vi "SplitSignals.vi"(0 "VI reference":refnum<vi>, 1 "Filename":path=path "E:/LabVIEW/Data/Test Data/Subj-Austin_Trial-1_Condition-None.lvm", 11 "Error In":errorcluster) -> (2 "EGG":dynamicdata(graph), 3 "Filename Out":path=path "E:/LabVIEW/Data/Test Data/Subj-Austin_Trial-1_Condition-None.lvm" caption="Filename", 4 "Flow":dynamicdata(graph), 6 "Pressure":dynamicdata(graph), 8 "Audio":dynamicdata(graph), 10 "SPL":dynamicdata(graph), 14 "Upper SPL":dbl, 15 "Error Out":errorcluster)   [LabVIEW 2019, in "AnalysisSupport.lvlib"]
uses:
  AnalysisSupport.lvlib
panel:
  out "Signals (Array)":string[](array[string])
  out "Comment":string
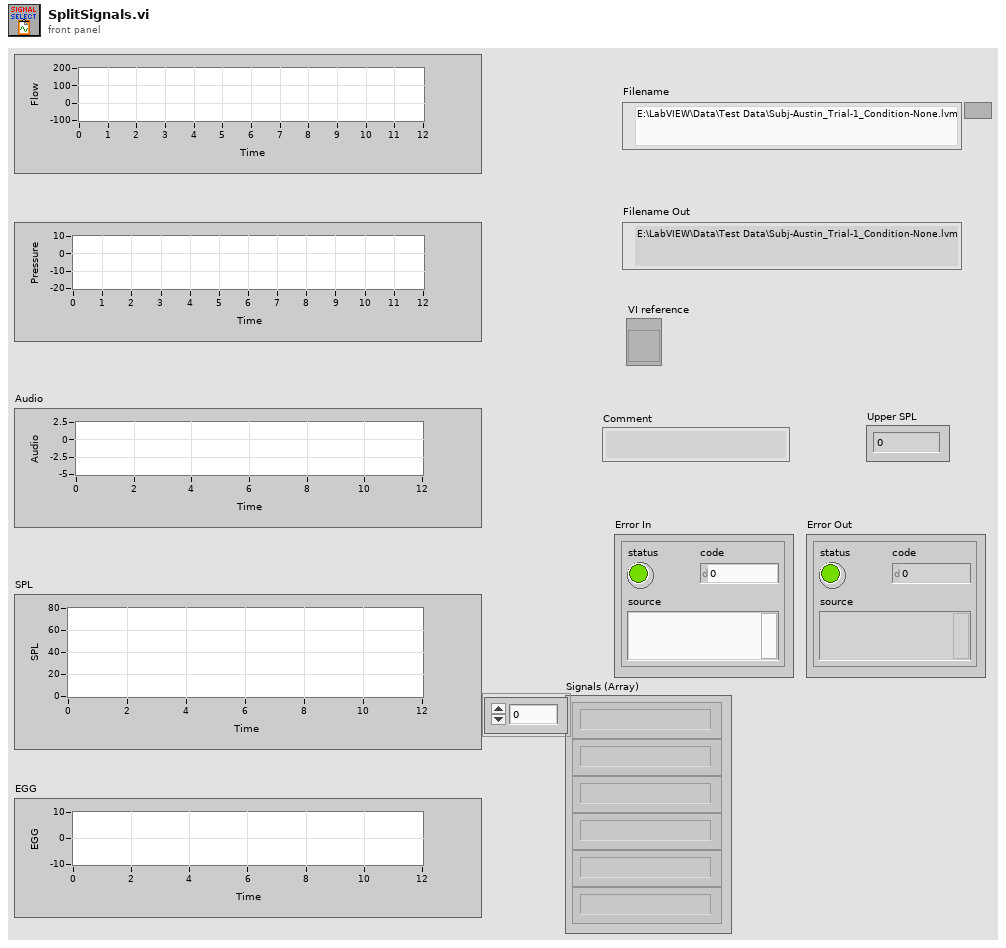
[diagram p1: front panel]
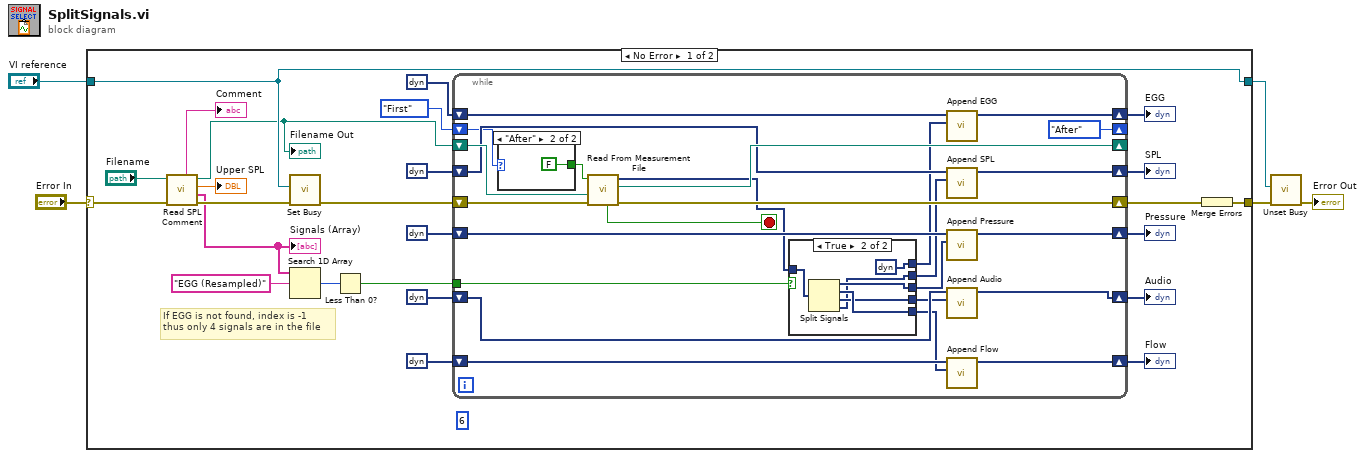
[diagram p0: block diagram]
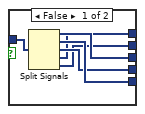
[diagram p2: hidden frame]
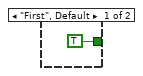
[diagram p3: hidden frame]
diagram:
  n1 = case shown="No Error" "Error In" {
    selector: "Error In" -> [w9 w71]
    tunnel: [w30 w71] -> w4
    tunnel: "VI reference" -> [w18 w70]
    tunnel: [w18 w70] -> w1
    frame No Error {
      (unwired) 6
      # "If EGG is not found, index is -1\nthus only 4 signals are in the file"
      n2 = call "Read SPL Comment.vi"("error in (no error)"=w9, "Filename"="Filename") -> ("error out"=w10:errorcluster, "Signals"=w6:string[], "Upper SPL"=→"Upper SPL":dbl, "Filename Out"=w14:path, "Comment"=→"Comment":string)  [unwired: 5 in]
      "Filename Out" <- w14
      "Signals (Array)" <- w6
      n3 = call <vilib>:"Set Busy.vi"("error in (no error)"=w10, "VI reference (current VI)"=w18) -> ("error out"=w7:errorcluster)  [unwired: 8 in, 1 out]
      n4 = Search 1D Array(1D array=w6, element="EGG (Resampled)") -> (index of element=w12:i32)  [unwired: 1 in]
      n5 = Less Than 0?(x=w12) -> (x < 0?=w11:bool)
      n6 = while {
        shift-right: [w54] -> w22
        shift-left: w7 -> [w53]
        shift-right: [w55] -> _
        shift-left: w14 -> [w52]
        shift-right: [w43] -> w25
        shift-left: dynamicdata [] ("Waveform Graph") -> [w50]
        shift-right: [w39] -> w21
        shift-left: dynamicdata [] ("Waveform Graph") -> [w49]
        shift-right: [w42] -> w24
        shift-left: dynamicdata [] ("Waveform Graph") -> [w48]
        shift-right: [w40] -> w23
        shift-left: dynamicdata [] ("Waveform Graph") -> [w47]
        shift-right: [enum16{"First", "After"}."After"] -> _
        shift-left: enum16{"First", "After"}."First" -> [w38]
        shift-right: [w32] -> w16
        shift-left: dynamicdata [] ("Waveform Graph") -> [w33]
        tunnel: w11 -> [w31]
        stop <- w51 stop-if-true
        n7 = case shown="\"After\"" w38 {
          tunnel: [TRUE ("Reset") FALSE ("Reset")] -> w37
          frame "First", Default {
          }
          frame "After" {
          }
        }
        n8 = call "Read From Measurement File"("error in (no error)"=w53, "Filename"=w52, "Reset"=w37) -> ("error out"=w54:errorcluster, "Filename Out"=w55:path, "Signals"=w41:dynamicdata, "EOF?"=w51:bool)  [unwired: 3 in, 2 out]
        n9 = case shown="True" w31 {
          tunnel: [w61 w65] -> w46
          tunnel: [w60 w64] -> w45
          tunnel: [w59 w63] -> w44
          tunnel: w41 -> [w58 w67]
          tunnel: [w57 w62] -> w35
          tunnel: [w56 dynamicdata [] ("Waveform Graph")] -> w34
          frame False {
            n10 = Split Signals(w58) -> (w61:dynamicdata, w60:dynamicdata, w59:dynamicdata, w56:dynamicdata, w57:dynamicdata)  [unwired: 5 in]
          }
          frame True {
            n11 = Split Signals(w67) -> (w65:dynamicdata, w64:dynamicdata, w63:dynamicdata, w62:dynamicdata)  [unwired: 4 in]
          }
        }
        n12 = call "Append EGG"("Input Signal B"=w34, "Input Signal A"=w33) -> ("Appended Signals"=w32:dynamicdata)  [unwired: 8 in, 1 out]
        n13 = call "Append SPL"("Input Signal B"=w35, "Input Signal A"=w47) -> ("Appended Signals"=w40:dynamicdata)  [unwired: 8 in, 1 out]
        n14 = call "Append Pressure"("Input Signal B"=w46, "Input Signal A"=w50) -> ("Appended Signals"=w43:dynamicdata)  [unwired: 8 in, 1 out]
        n15 = call "Append Audio"("Input Signal B"=w44, "Input Signal A"=w48) -> ("Appended Signals"=w42:dynamicdata)  [unwired: 8 in, 1 out]
        n16 = call "Append Flow"("Input Signal B"=w45, "Input Signal A"=w49) -> ("Appended Signals"=w39:dynamicdata)  [unwired: 8 in, 1 out]
      }
      "Flow" <- w21
      "Pressure" <- w25
      "SPL" <- w23
      "Audio" <- w24
      "EGG" <- w16
      n17 = Merge Errors(w22) -> (w30:errorcluster)
    }
    frame Error {
    }
  }
  n18 = call <vilib>:"Unset Busy.vi"("error in (no error)"=w4, "VI reference (current VI)"=w1) -> ("error out"=→"Error Out":errorcluster)  [unwired: 9 in]
